vi "Log State.vi"(8 "error in":errorcluster, 10 "Model Status":T3, 11 "Data":T1) -> (0 "error out":errorcluster, 3 "Data out":T1)   [LabVIEW 2015, in "Logger.lvlib"]
uses:
  Logger.lvlib
  Model/TypeDefs/Get Model Status Control.ctl
  TypeDefs/Logger Data.ctl
  TypeDefs/Logger State.ctl
  Model/Model.lvlib
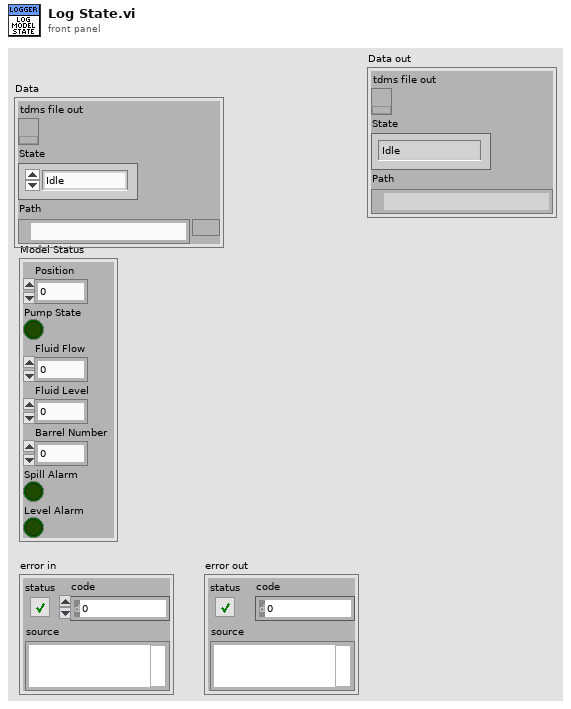
[diagram p1: front panel]
types:
  T1 = typedef "Logger.lvlib/Logger Data.ctl" = cluster{"tdms file out":refnum<k34>, "State":T2, "Path":path}
  T2 = typedef "Logger.lvlib/Logger State.ctl" = enum16{"Idle", "Working"}
  T3 = typedef "Model.lvlib/Get Model Status Control.ctl" = cluster{"Position":dbl, "Pump State":bool, "Fluid Flow":dbl, "Fluid Level":dbl, "Barrel Number":i32, "Spill Alarm":bool, "Level Alarm":bool}
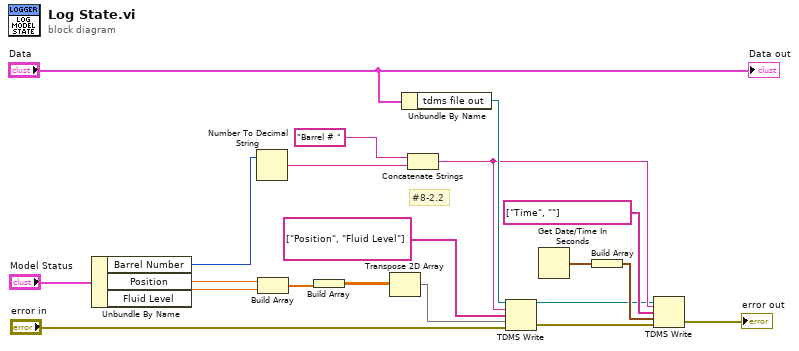
[diagram p0: block diagram]
diagram:
  # "#8-2.2"
  n1 = Unbundle By Name("Model Status") -> ("Barrel Number"=w17:i32, "Position"=w19:dbl, "Fluid Level"=w18:dbl)
  n2 = Number To Decimal String(number=w17) -> (decimal integer string=w6:string)  [unwired: 1 in]
  n3 = Build Array(w19, w18) -> (w10:dbl[])
  n4 = Build Array(w10) -> (w9:dbl[][])
  n5 = Transpose 2D Array(2D array=w9) -> (transposed array=w8:dbl[][])
  n6 = Unbundle By Name("Data") -> ("tdms file out"=w13:refnum<k34>)
  n7 = Concatenate Strings("Barrel # " ("string"), w6) -> (w4:string)
  n8 = TDMS Write(0:w13, 5:w4, 7:string[] ["Position", "Fluid Level"], 9:w8, 11:"error in") -> (4:w1:refnum<k34>, 15:w15:errorcluster)  [unwired: 1 in, 2 out]
  n9 = Get Date/Time In Seconds() -> (seconds since 1Jan1904=w12:timestamp)
  n10 = Build Array(w12) -> (w11:timestamp[])
  n11 = TDMS Write(0:w1, 5:w4, 7:string[] ["Time", ""], 9:w11, 11:w15) -> (15:→"error out":errorcluster)  [unwired: 1 in, 3 out]
  "Data out" <- "Data"
